vi "RSNRPZ Set Source Gamma Magnitude.vi"(8 "error in (no error)":errorcluster, 9 "Magnitude (1.0)":dbl=1.0 format="%.2p", 10 "Channel (1)":i32=1, 11 "VISA session":refnum<visa-resource-name> caption="VISA resource name") -> (0 "error out":errorcluster, 3 "dup VISA session":refnum<visa-resource-name> caption="VISA resource name")   [LabVIEW 2010]
doc: "This VI sets the magnitude of the reflection coefficient for measured-value correction.\n\nRemote-control command(s):\nSENS:SGAM:MAGN"
uses:
  rsnrpz_32.dll
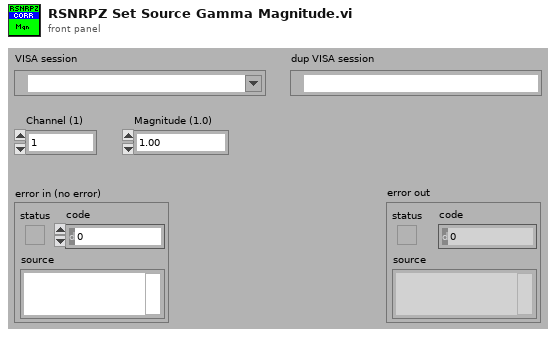
[diagram p1: front panel]
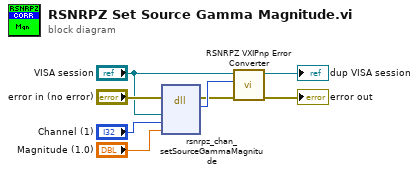
[diagram p0: block diagram]
diagram:
  n1 = dll-call lib="rsnrpz_32.dll" fn="rsnrpz_chan_setSourceGammaMagnitude"(error in="error in (no error)", "VISA Session"="VISA session", "Channel"="Channel (1)", "Magnitude"="Magnitude (1.0)") -> (error out=w5:errorcluster, "Status"=w8:i32)  [unwired: 5 in, 1 out]
  n2 = call <instrlib>:"RSNRPZ VXIPnp Error Converter.vi"("error in"=w5, "VXIPnp error code"=w8, "VISA session"="VISA session") -> ("error out"=→"error out":errorcluster, "dup VISA session"=→"dup VISA session":refnum<visa-resource-name>)  [unwired: 7 in]
